vi "Update Run Config.vi"(8 "error in (no error)":errorcluster, 10 "Run config file":path, 11 "Guardian in":refnum<class "Guardian.lvclass">) -> (0 "error out":errorcluster, 3 "Guardian out":refnum<class "Guardian.lvclass">)   [LabVIEW 2020, in "TALOS.lvlib" / "Guardian.lvlib" / "Guardian.lvclass"]
uses:
  Guardian.lvclass
  Guardian.lvclass/Guardian.ctl
  TALOS.lvlib
  Classes/uService List/uService List.lvclass
  fcb3572a-2cec-4fc7-ae89-858ca11508d7.vi
  24f5ad44-0365-4765-b898-cef69fd9b7bb.vi
  Guardian Messages/Launch uService Msg/Launch uService Msg.lvclass
  Guardian Messages/Kill uService Msg/Kill uService Msg.lvclass
  builds/Actor Framework PPL/Actor Framework.lvlibp/1abvi3w/vi.lib/ActorFramework/Actor/Actor.lvclass
  C:/Users/marco/Documents/GitHub_Lab/TALOS/talos/Ancestor/Ancestor/Ancestor.lvclass
  C:/Users/marco/Documents/GitHub_Lab/TALOS/builds/Actor Framework PPL/Actor Framework.lvlibp/1abvi3w/vi.lib/ActorFramework/Actor/Actor.lvclass
  C:/Users/marco/Documents/GitHub_Lab/TALOS/talos/Guardian/Guardian/Guardian.lvclass
  Classes/uService List/Get all IDs.vi
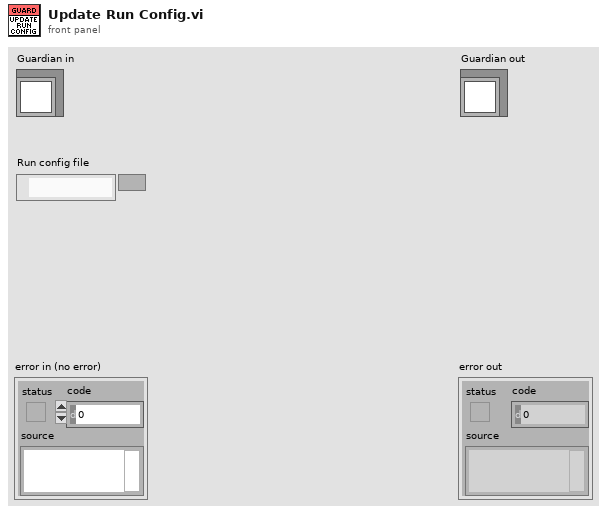
[diagram p1: front panel]
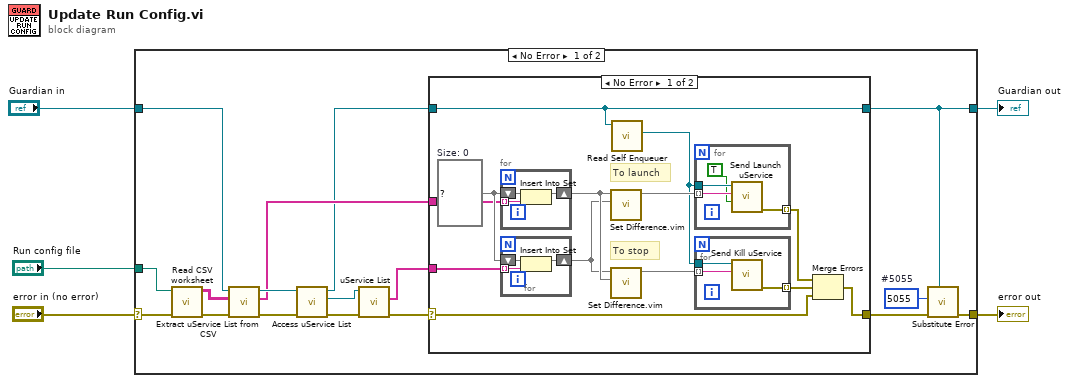
[diagram p0: block diagram]
diagram:
  n1 = case shown="No Error" "error in (no error)" {
    selector: "error in (no error)" -> [w21 w52]
    tunnel: [w8 w52] -> w4
    tunnel: [w7 w51] -> w2
    tunnel: "Guardian in" -> [w18 w51]
    tunnel: "Run config file" -> [w22 _]
    frame No Error {
      w6 = 5055  # #5055
      n2 = call "Read CSV worksheet.vi"("error in (no error)"=w21, "appended path"=w22) -> ("error out"=w20:errorcluster, "Sheet"=w19:string[][])  [unwired: 8 in]
      n3 = call "Extract uService List from CSV.vi"("error in (no error)"=w20, "CSV table"=w19, "Guardian in"=w18) -> ("error out"=w15:errorcluster, "uS array"=w13:string[], "Guardian out"=w16:refnum<class "Guardian.lvclass">)  [unwired: 6 in]
      n4 = call-dynamic "Access uService List.vi"("error in (no error)"=w15, "Ancestor in"=w16) -> ("error out"=w14:errorcluster, "uService List out"=w17:refnum<class "uService List.lvclass">, "Ancestor out"=w11:refnum<class "Guardian.lvclass">)  [unwired: 7 in]
      n5 = call-poly "uService List.vi"("error in (no error)"=w14, "uService List"=w17) -> ("error out"=w10:errorcluster, "All IDs"=w12:string[])  [unwired: 7 in, 1 out]
      n6 = case shown="No Error" w10 {
        selector: w10 -> [w24 w50]
        tunnel: w13 -> [w32 _]
        tunnel: w12 -> [w30 _]
        tunnel: w11 -> [w28 w49]
        tunnel: [w23 w50] -> w9
        tunnel: [w28 w49] -> w7
        frame No Error {
          w33 = set{string} {}  # Size: 0
          # "To stop"
          # "To launch"
          n7 = for {
            shift-right: [w41] -> w31
            shift-left: w33 -> [w40]
            tunnel: w32 -> [w39] mode=indexing
            n8 = Insert Into Set(10:w39, 11:w40) -> (3:w41:set{string})  [unwired: 1 out]
          }
          n9 = for {
            shift-right: [w38] -> w29
            shift-left: w33 -> [w37]
            tunnel: w30 -> [w36] mode=indexing
            n10 = Insert Into Set(10:w36, 11:w37) -> (3:w38:set{string})  [unwired: 1 out]
          }
          n11 = call "Set Difference.vim"("set 2"=w29, "set 1"=w31) -> ("difference"=w35:set{string})  [unwired: 9 in]
          n12 = call "Set Difference.vim"("set 2"=w31, "set 1"=w29) -> ("difference"=w34:set{string})  [unwired: 9 in]
          n13 = call "Read Self Enqueuer.vi"("Actor"=w28) -> ("Self Enqueuer"=w27:refnum<class "Message Enqueuer.lvclass">)  [unwired: 10 in]
          n14 = for {
            tunnel: w35 -> [w47] mode=indexing
            tunnel: w27 -> [w48]
            tunnel: [w45] -> w26 mode=indexing
            n15 = call "Send Launch uService.vi"("GUI?"=TRUE, "uService Class Name"=w47, "Message Enqueuer"=w48) -> ("error out"=w45:errorcluster)  [unwired: 7 in, 1 out]
          }
          n16 = for {
            tunnel: w34 -> [w44] mode=indexing
            tunnel: w27 -> [w43]
            tunnel: [w42] -> w25 mode=indexing
            n17 = call "Send Kill uService.vi"("uService"=w44, "Message Enqueuer"=w43) -> ("error out"=w42:errorcluster)  [unwired: 8 in, 1 out]
          }
          n18 = Merge Errors(w26, w25, w24) -> (w23:errorcluster)
        }
        frame Error {
        }
      }
      n19 = call "Substitute Error.vi"("LabVIEW Object"=w7, "error in (no error)"=w9, "Error Code"=w6) -> ("error out"=w8:errorcluster)  [unwired: 8 in]
    }
    frame Error {
    }
  }
  "error out" <- w4
  "Guardian out" <- w2
